vi "Configure_Transfer_SMUs.vi"(6 "Var2 step settings":T3, 8 "error in (no error)":errorcluster, 9 "Var1 sweep settings":T2, 10 "SMU Config":T1, 11 "VISA In":refnum<visa-resource-name>) -> (0 "error out":errorcluster, 3 "VISA Out":refnum<visa-resource-name>)   [LabVIEW 2012]
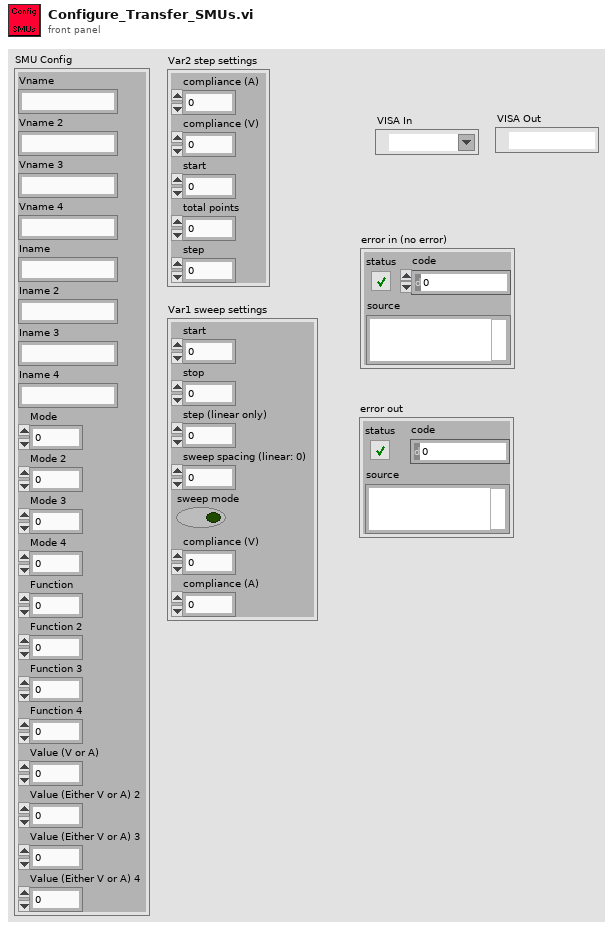
[diagram p1: front panel]
types:
  T1 = cluster{"Vname":string, "Vname 2":string, "Vname 3":string, "Vname 4":string, "Iname":string, "Iname 2":string, "Iname 3":string, "Iname 4":string, "Mode":u16, "Mode 2":u16, "Mode 3":u16, "Mode 4":u16, "Function":u16, "Function 2":u16, "Function 3":u16, "Function 4":u16, "Value (V or A)":dbl, "Value (Either V or A) 2":dbl, "Value (Either V or A) 3":dbl, "Value (Either V or A) 4":dbl}
  T2 = cluster{"start":dbl, "stop":dbl, "step (linear only)":dbl, "sweep spacing (linear: 0)":u16, "sweep mode":bool, "compliance (V)":dbl, "compliance (A)":dbl}
  T3 = cluster{"compliance (A)":dbl, "compliance (V)":dbl, "start":dbl, "total points":u16, "step":dbl}
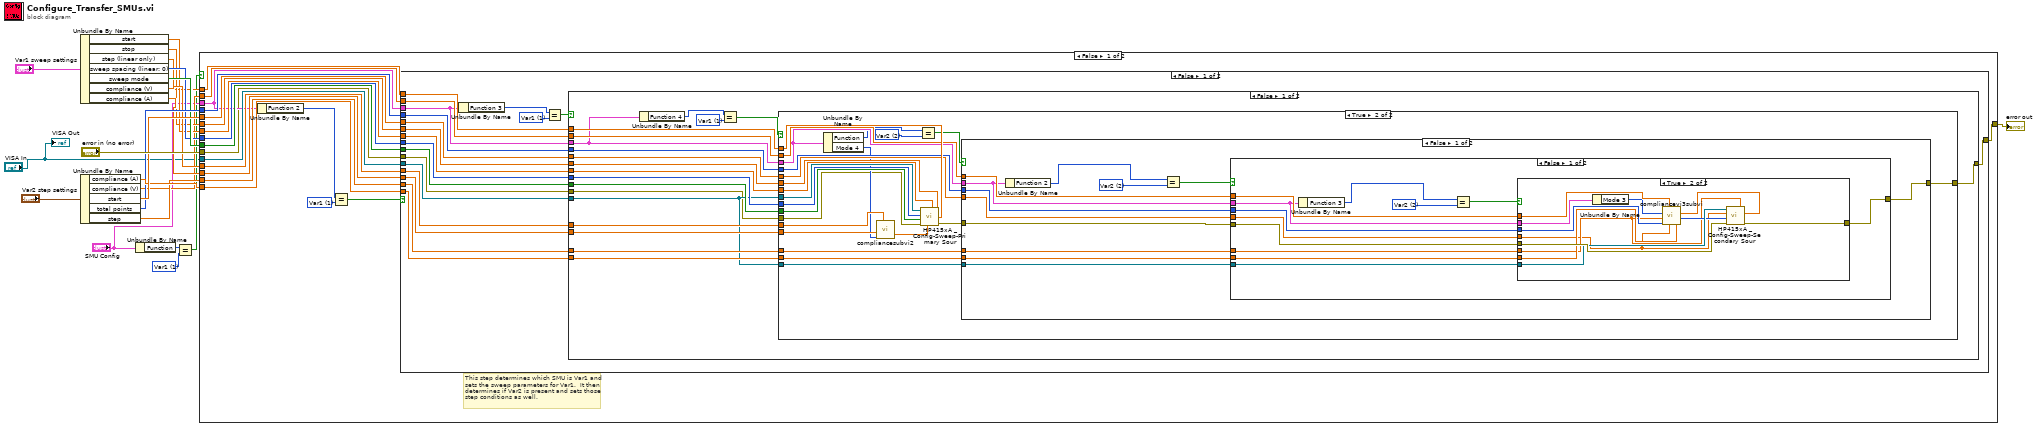
[diagram p0: block diagram]
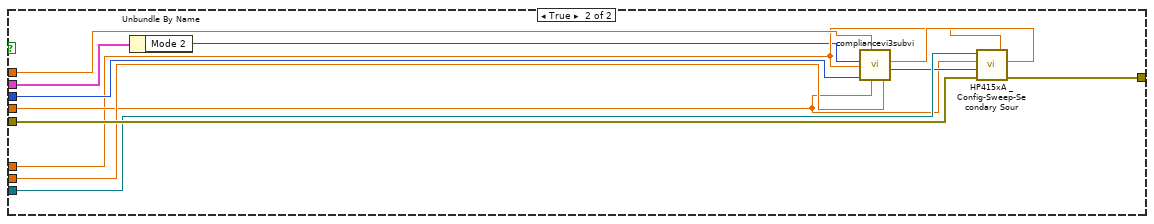
[diagram p4: hidden frame]
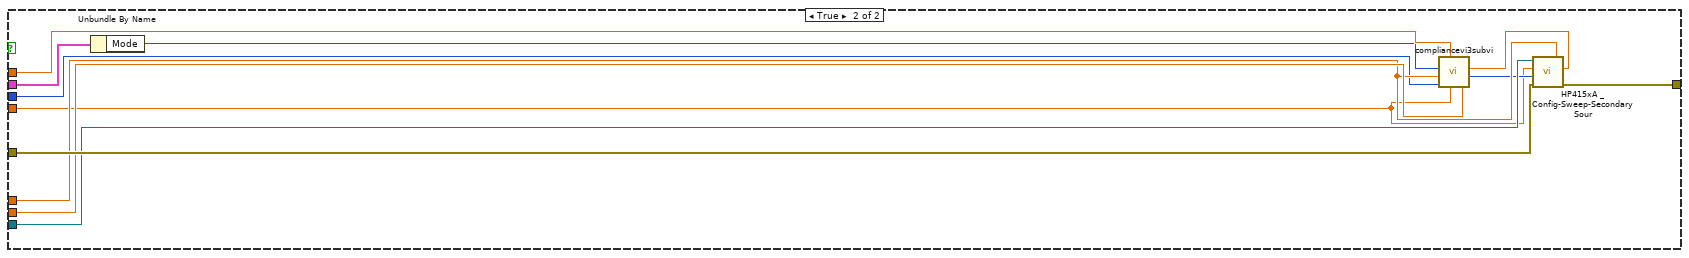
[diagram p5: hidden frame]
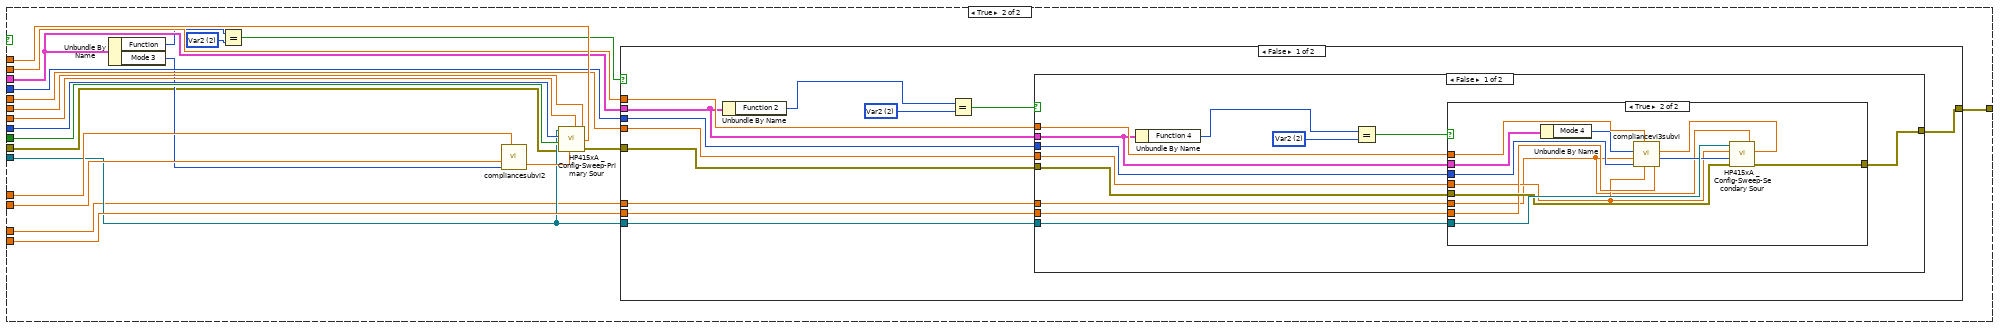
[diagram p6: hidden frame]
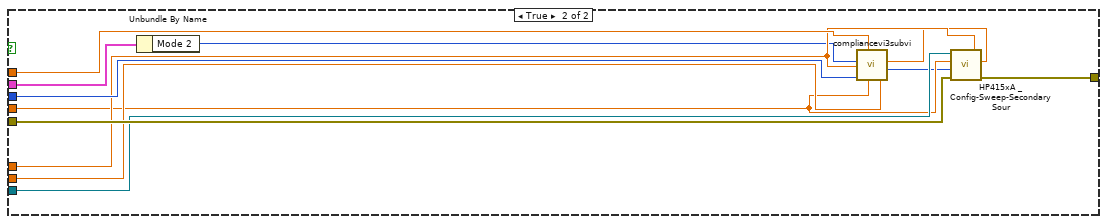
[diagram p8: hidden frame]
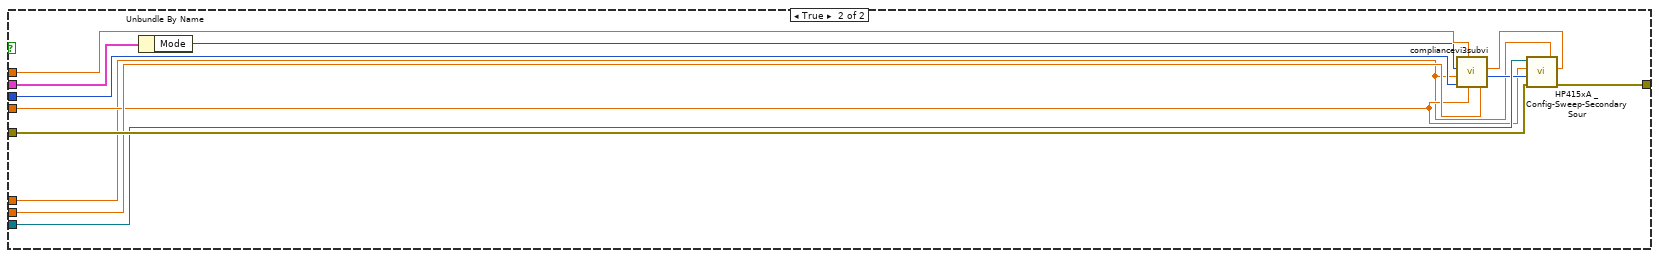
[diagram p9: hidden frame]
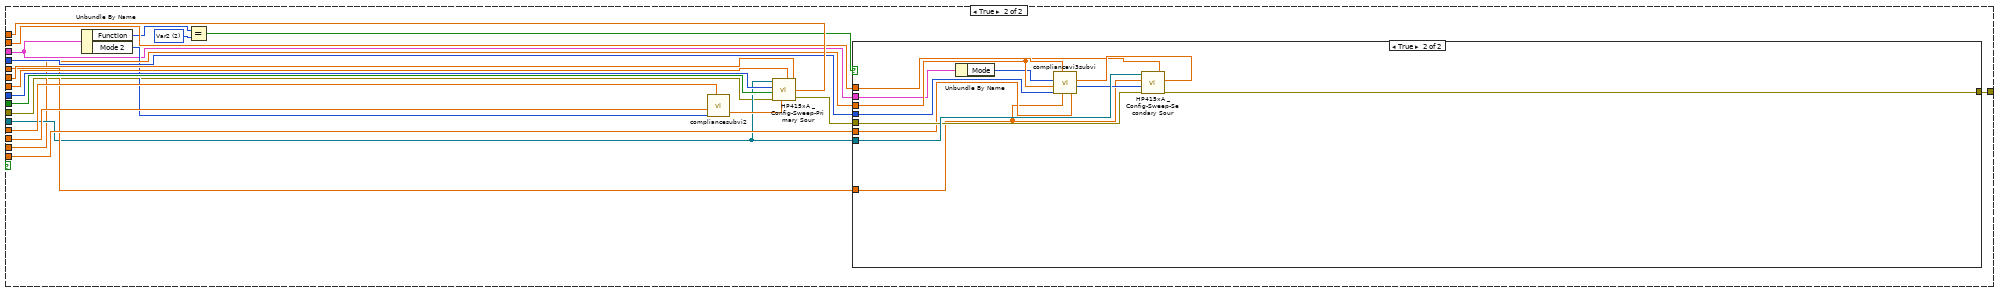
[diagram p10: hidden frame]
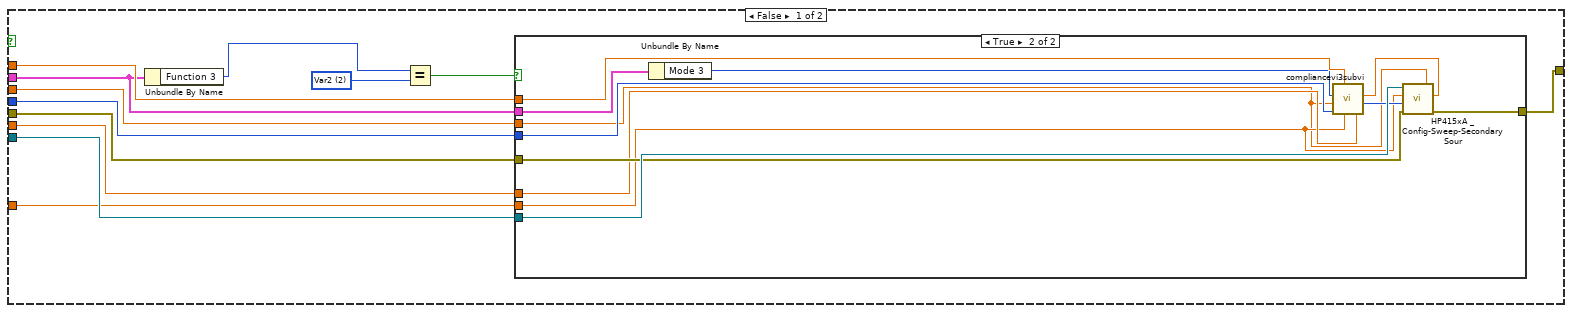
[diagram p11: hidden frame]
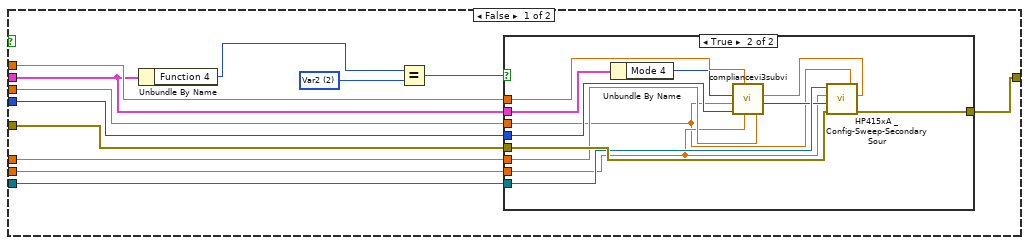
[diagram p12: hidden frame]
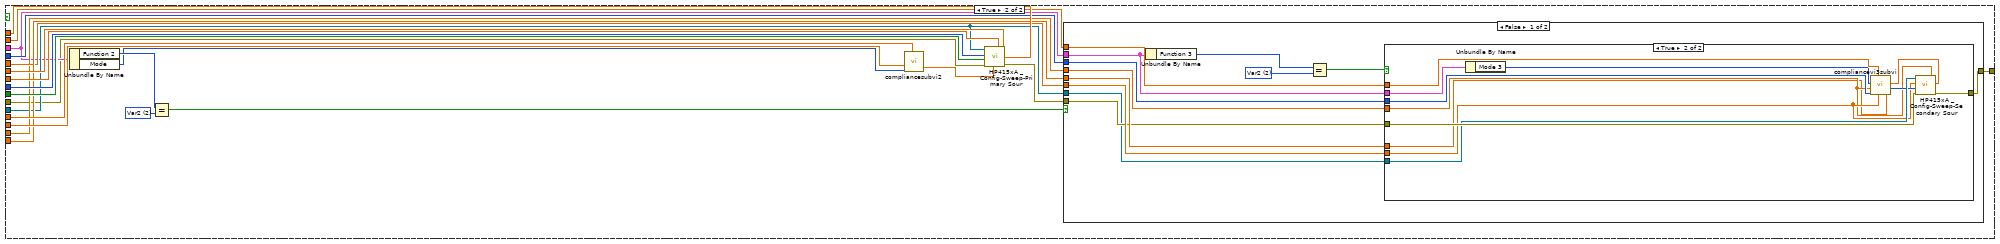
[diagram p14: hidden frame]
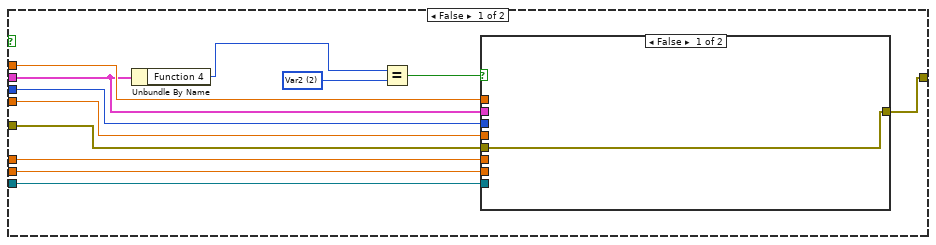
[diagram p15: hidden frame]
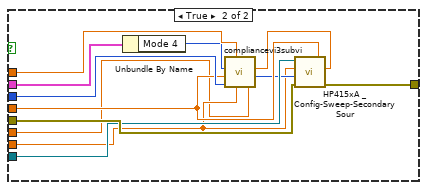
[diagram p16: hidden frame]
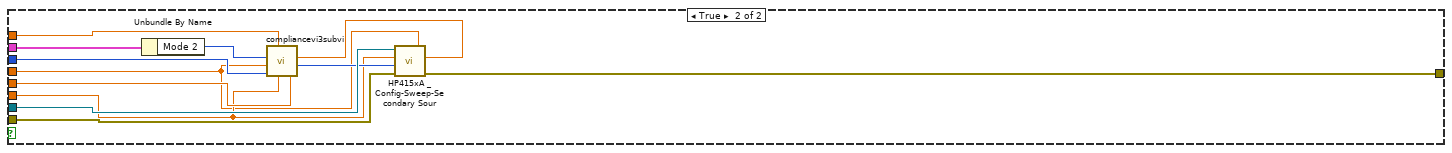
[diagram p17: hidden frame]
diagram:
  w2 = u16 1 items=["disabled", "Var1", "Var2", "Var1'", "Constant"] ("Function")
  n1 = Unbundle By Name("Var1 sweep settings") -> ("start"=w11:dbl, "stop"=w10:dbl, "step (linear only)"=w7:dbl, "sweep spacing (linear: 0)"=w12:u16, "sweep mode"=w13:bool, "compliance (V)"=w14:dbl, "compliance (A)"=w15:dbl)
  n2 = Unbundle By Name("Var2 step settings") -> ("compliance (A)"=w18:dbl, "compliance (V)"=w9:dbl, "start"=w19:dbl, "total points"=w16:u16, "step"=w17:dbl)
  n3 = Unbundle By Name("SMU Config") -> ("Function"=w4:u16)
  n4 = Equal?(x=w4, y=w2) -> (x = y?=w3:bool)
  n5 = case shown="False" w3 {
    tunnel: w14 -> [w38 w350]
    tunnel: w15 -> [w39 w349]
    tunnel: w12 -> [w36 w348]
    tunnel: w13 -> [w37 w347]
    tunnel: w7 -> [w33 w346]
    tunnel: w10 -> [w32 w345]
    tunnel: w11 -> [w34 w344]
    tunnel: "VISA In" -> [w35 w335]
    tunnel: w18 -> [w30 w341]
    tunnel: w9 -> [w29 w340]
    tunnel: w19 -> [w28 w339]
    tunnel: w16 -> [w27 w338]
    tunnel: w17 -> [w26 w337]
    tunnel: "SMU Config" -> [w25 w332]
    tunnel: [w23 w331] -> w20
    tunnel: "error in (no error)" -> [w22 w330]
    frame False {
      w40 = u16 1 items=["disabled", "Var1", "Var2", "Var1'", "Constant"] ("Function")
      # "This step determines which SMU is Var1 and\nsets the sweep parameters for Var1.  It then\ndetermines if Var2 is present and sets those\nstep conditions as well."
      n6 = Unbundle By Name(w25) -> ("Function 2"=w24:u16)
      n7 = Equal?(x=w24, y=w40) -> (x = y?=w31:bool)
      n8 = case shown="False" w31 {
        tunnel: w39 -> [w50 w267]
        tunnel: w38 -> [w51 w266]
        tunnel: w37 -> [w52 w265]
        tunnel: w36 -> [w53 w264]
        tunnel: w35 -> [w57 w255]
        tunnel: w34 -> [w56 w263]
        tunnel: w33 -> [w54 w262]
        tunnel: w32 -> [w55 w261]
        tunnel: w30 -> [w49 w258]
        tunnel: w29 -> [w48 w257]
        tunnel: w28 -> [w46 w256]
        tunnel: w27 -> [w47 w253]
        tunnel: w26 -> [w45 w252]
        tunnel: w25 -> [w44 w249]
        tunnel: [w42 w248] -> w23
        tunnel: w22 -> [w41 w247]
        frame False {
          w59 = u16 1 items=["disabled", "Var1", "Var2", "Var1'", "Constant"] ("Function")
          n9 = Unbundle By Name(w44) -> ("Function 3"=w43:u16)
          n10 = Equal?(x=w43, y=w59) -> (x = y?=w58:bool)
          n11 = case shown="False" w58 {
            tunnel: w57 -> [w64 w171]
            tunnel: w56 -> [w76 w185]
            tunnel: w55 -> [w73 w184]
            tunnel: w54 -> [w72 w183]
            tunnel: w53 -> [w75 w182]
            tunnel: w52 -> [w74 w181]
            tunnel: w51 -> [w71 w180]
            tunnel: w50 -> [w70 w179]
            tunnel: w49 -> [w69 w175]
            tunnel: w48 -> [w68 w174]
            tunnel: w47 -> [w67 w173]
            tunnel: w46 -> [w66 w170]
            tunnel: w45 -> [w65 w169]
            tunnel: w44 -> [w62 w168]
            tunnel: [w61 w165] -> w42
            tunnel: w41 -> [w60 w164]
            frame False {
              w78 = u16 1 items=["disabled", "Var1", "Var2", "Var1'", "Constant"] ("Function")
              n12 = Unbundle By Name(w62) -> ("Function 4"=w63:u16)
              n13 = Equal?(x=w63, y=w78) -> (x = y?=w77:bool)
              n14 = case shown="True" w77 {
                tunnel: w76 -> [_ w101]
                tunnel: w64 -> [_ w100]
                tunnel: w75 -> [_ w99]
                tunnel: w74 -> [_ w98]
                tunnel: w73 -> [_ w97]
                tunnel: w72 -> [_ w96]
                tunnel: w71 -> [_ w95]
                tunnel: w70 -> [_ w94]
                tunnel: w69 -> [_ w91]
                tunnel: w68 -> [_ w90]
                tunnel: w67 -> [_ w89]
                tunnel: w66 -> [_ w88]
                tunnel: w65 -> [_ w87]
                tunnel: w64 -> [_ w85]
                tunnel: w62 -> [_ w84]
                tunnel: [w79 w81] -> w61
                tunnel: w60 -> [w79 w80]
                frame False {
                }
                frame True {
                  w93 = u16 2 items=["disabled", "Var1", "Var2", "Var1'", "Constant"] ("Function")
                  n15 = Unbundle By Name(w84) -> ("Function"=w83:u16, "Mode 4"=w82:u16)
                  n16 = call "compliancesubvi2.vi"("compliance (V)"=w95, "Mode"=w82, "compliance (A)"=w94) -> ("compliance"=w102:dbl)  [unwired: 3 in, 1 out]
                  n17 = Equal?(x=w83, y=w93) -> (x = y?=w92:bool)
                  n18 = call "HP415xA _Config-Sweep-Primary Sour.vi"("step (linear only)"=w96, "stop"=w97, "start"=w101, "compliance"=w102, "error in (no error)"=w80, "sweep mode"=w98, "sweep spacing (linear: 0)"=w99, "VISA session"=w100) -> ("error out"=w86:errorcluster)  [unwired: 2 in]
                  n19 = case shown="False" w92 {
                    tunnel: w91 -> [w112 w161]
                    tunnel: w90 -> [w111 w156]
                    tunnel: w89 -> [w110 w155]
                    tunnel: w88 -> [w109 w157]
                    tunnel: w87 -> [w108 w160]
                    tunnel: w86 -> [w107 w163]
                    tunnel: w85 -> [w106 w162]
                    tunnel: w84 -> [w104 w154]
                    tunnel: [w103 w152] -> w81
                    frame False {
                      w114 = u16 2 items=["disabled", "Var1", "Var2", "Var1'", "Constant"] ("Function")
                      n20 = Unbundle By Name(w104) -> ("Function 2"=w105:u16)
                      n21 = Equal?(x=w105, y=w114) -> (x = y?=w113:bool)
                      n22 = case shown="False" w113 {
                        tunnel: w112 -> [w124 w148]
                        tunnel: w111 -> [w123 w149]
                        tunnel: w110 -> [w122 w147]
                        tunnel: w109 -> [w121 w145]
                        tunnel: w108 -> [w120 w143]
                        tunnel: w107 -> [w119 w151]
                        tunnel: w106 -> [w118 w150]
                        tunnel: w104 -> [w116 w142]
                        tunnel: [w115 w140] -> w103
                        frame False {
                          w126 = u16 2 items=["disabled", "Var1", "Var2", "Var1'", "Constant"] ("Function")
                          n23 = Unbundle By Name(w116) -> ("Function 3"=w117:u16)
                          n24 = Equal?(x=w117, y=w126) -> (x = y?=w125:bool)
                          n25 = case shown="True" w125 {
                            tunnel: w124 -> [_ w135]
                            tunnel: w123 -> [_ w136]
                            tunnel: w122 -> [_ w137]
                            tunnel: w121 -> [_ w131]
                            tunnel: w120 -> [_ w132]
                            tunnel: w119 -> [w127 w139]
                            tunnel: w118 -> [_ w138]
                            tunnel: w116 -> [_ w130]
                            tunnel: [w127 w128] -> w115
                            frame False {
                            }
                            frame True {
                              n26 = Unbundle By Name(w130) -> ("Mode 3"=w129:u16)
                              n27 = call "compliancevi3subvi.vi"("compliance (A)"=w135, "start"=w131, "compliance (V)"=w136, "total points"=w137, "step"=w132, "Mode"=w129) -> ("total points 2"=w134:u16, "compliance"=w133:dbl)  [unwired: 1 in, 1 out]
                              n28 = call "HP415xA _Config-Sweep-Secondary Sour.vi"("compliance"=w133, "step"=w132, "error in (no error)"=w139, "total points"=w134, "start"=w131, "VISA session"=w138) -> ("error out"=w128:errorcluster)  [unwired: 1 in]
                            }
                          }
                        }
                        frame True {
                          n29 = Unbundle By Name(w142) -> ("Mode 2"=w141:u16)
                          n30 = call "compliancevi3subvi.vi"("compliance (A)"=w148, "start"=w145, "compliance (V)"=w149, "total points"=w147, "step"=w143, "Mode"=w141) -> ("total points 2"=w146:u16, "compliance"=w144:dbl)  [unwired: 1 in, 1 out]
                          n31 = call "HP415xA _Config-Sweep-Secondary Sour.vi"("compliance"=w144, "step"=w143, "error in (no error)"=w151, "total points"=w146, "start"=w145, "VISA session"=w150) -> ("error out"=w140:errorcluster)  [unwired: 1 in]
                        }
                      }
                    }
                    frame True {
                      n32 = Unbundle By Name(w154) -> ("Mode"=w153:u16)
                      n33 = call "compliancevi3subvi.vi"("compliance (A)"=w161, "start"=w157, "compliance (V)"=w156, "total points"=w155, "step"=w160, "Mode"=w153) -> ("total points 2"=w158:u16, "compliance"=w159:dbl)  [unwired: 1 in, 1 out]
                      n34 = call "HP415xA _Config-Sweep-Secondary Sour.vi"("compliance"=w159, "step"=w160, "error in (no error)"=w163, "total points"=w158, "start"=w157, "VISA session"=w162) -> ("error out"=w152:errorcluster)  [unwired: 1 in]
                    }
                  }
                }
              }
            }
            frame True {
              w177 = u16 2 items=["disabled", "Var1", "Var2", "Var1'", "Constant"] ("Function")
              n35 = Unbundle By Name(w168) -> ("Function"=w167:u16, "Mode 3"=w166:u16)
              n36 = Equal?(x=w167, y=w177) -> (x = y?=w176:bool)
              n37 = call "compliancesubvi2.vi"("compliance (V)"=w180, "Mode"=w166, "compliance (A)"=w179) -> ("compliance"=w178:dbl)  [unwired: 3 in, 1 out]
              n38 = call "HP415xA _Config-Sweep-Primary Sour.vi"("step (linear only)"=w183, "stop"=w184, "start"=w185, "compliance"=w178, "error in (no error)"=w164, "sweep mode"=w181, "sweep spacing (linear: 0)"=w182, "VISA session"=w171) -> ("error out"=w172:errorcluster)  [unwired: 2 in]
              n39 = case shown="False" w176 {
                tunnel: w175 -> [w193 w244]
                tunnel: w174 -> [w192 w243]
                tunnel: w173 -> [w190 w242]
                tunnel: w172 -> [w195 w246]
                tunnel: w171 -> [w194 w245]
                tunnel: w170 -> [w189 w239]
                tunnel: w169 -> [w191 w238]
                tunnel: w168 -> [w188 w237]
                tunnel: [w186 w235] -> w165
                frame False {
                  w197 = u16 2 items=["disabled", "Var1", "Var2", "Var1'", "Constant"] ("Function")
                  n40 = Unbundle By Name(w188) -> ("Function 2"=w187:u16)
                  n41 = Equal?(x=w187, y=w197) -> (x = y?=w196:bool)
                  n42 = case shown="False" w196 {
                    tunnel: w195 -> [w207 w234]
                    tunnel: w194 -> [w206 w233]
                    tunnel: w193 -> [w205 w230]
                    tunnel: w192 -> [w204 w231]
                    tunnel: w191 -> [w201 w229]
                    tunnel: w190 -> [w203 w232]
                    tunnel: w189 -> [w202 w228]
                    tunnel: w188 -> [w199 w225]
                    tunnel: [w198 w223] -> w186
                    frame False {
                      w209 = u16 2 items=["disabled", "Var1", "Var2", "Var1'", "Constant"] ("Function")
                      n43 = Unbundle By Name(w199) -> ("Function 4"=w200:u16)
                      n44 = Equal?(x=w200, y=w209) -> (x = y?=w208:bool)
                      n45 = case shown="True" w208 {
                        tunnel: w207 -> [w210 w221]
                        tunnel: w206 -> [_ w222]
                        tunnel: w205 -> [_ w219]
                        tunnel: w204 -> [_ w220]
                        tunnel: w203 -> [_ w218]
                        tunnel: w202 -> [_ w215]
                        tunnel: w201 -> [_ w214]
                        tunnel: w199 -> [_ w213]
                        tunnel: [w210 w211] -> w198
                        frame False {
                        }
                        frame True {
                          n46 = Unbundle By Name(w213) -> ("Mode 4"=w212:u16)
                          n47 = call "compliancevi3subvi.vi"("compliance (A)"=w219, "start"=w215, "compliance (V)"=w220, "total points"=w218, "step"=w214, "Mode"=w212) -> ("total points 2"=w217:u16, "compliance"=w216:dbl)  [unwired: 1 in, 1 out]
                          n48 = call "HP415xA _Config-Sweep-Secondary Sour.vi"("compliance"=w216, "step"=w214, "error in (no error)"=w221, "total points"=w217, "start"=w215, "VISA session"=w222) -> ("error out"=w211:errorcluster)  [unwired: 1 in]
                        }
                      }
                    }
                    frame True {
                      n49 = Unbundle By Name(w225) -> ("Mode 2"=w224:u16)
                      n50 = call "compliancevi3subvi.vi"("compliance (A)"=w230, "start"=w228, "compliance (V)"=w231, "total points"=w232, "step"=w229, "Mode"=w224) -> ("total points 2"=w227:u16, "compliance"=w226:dbl)  [unwired: 1 in, 1 out]
                      n51 = call "HP415xA _Config-Sweep-Secondary Sour.vi"("compliance"=w226, "step"=w229, "error in (no error)"=w234, "total points"=w227, "start"=w228, "VISA session"=w233) -> ("error out"=w223:errorcluster)  [unwired: 1 in]
                    }
                  }
                }
                frame True {
                  n52 = Unbundle By Name(w237) -> ("Mode"=w236:u16)
                  n53 = call "compliancevi3subvi.vi"("compliance (A)"=w244, "start"=w239, "compliance (V)"=w243, "total points"=w242, "step"=w238, "Mode"=w236) -> ("total points 2"=w241:u16, "compliance"=w240:dbl)  [unwired: 1 in, 1 out]
                  n54 = call "HP415xA _Config-Sweep-Secondary Sour.vi"("compliance"=w240, "step"=w238, "error in (no error)"=w246, "total points"=w241, "start"=w239, "VISA session"=w245) -> ("error out"=w235:errorcluster)  [unwired: 1 in]
                }
              }
            }
          }
        }
        frame True {
          w260 = u16 2 items=["disabled", "Var1", "Var2", "Var1'", "Constant"] ("Function")
          n55 = Unbundle By Name(w249) -> ("Function"=w251:u16, "Mode 2"=w250:u16)
          n56 = Equal?(x=w251, y=w260) -> (x = y?=w259:bool)
          n57 = call "compliancesubvi2.vi"("compliance (V)"=w266, "Mode"=w250, "compliance (A)"=w267) -> ("compliance"=w268:dbl)  [unwired: 3 in, 1 out]
          n58 = call "HP415xA _Config-Sweep-Primary Sour.vi"("step (linear only)"=w262, "stop"=w261, "start"=w263, "compliance"=w268, "error in (no error)"=w247, "sweep mode"=w265, "sweep spacing (linear: 0)"=w264, "VISA session"=w255) -> ("error out"=w254:errorcluster)  [unwired: 2 in]
          n59 = case shown="True" w259 {
            tunnel: w258 -> [w277 w326]
            tunnel: w257 -> [w276 w325]
            tunnel: w256 -> [w274 w321]
            tunnel: w255 -> [w279 w329]
            tunnel: w254 -> [w273 w328]
            tunnel: w253 -> [w275 w327]
            tunnel: w252 -> [w272 w323]
            tunnel: w249 -> [w271 w320]
            tunnel: [w269 w318] -> w248
            frame False {
              w280 = u16 2 items=["disabled", "Var1", "Var2", "Var1'", "Constant"] ("Function")
              n60 = Unbundle By Name(w271) -> ("Function 3"=w270:u16)
              n61 = Equal?(x=w270, y=w280) -> (x = y?=w278:bool)
              n62 = case shown="True" w278 {
                tunnel: w279 -> [w289 w317]
                tunnel: w277 -> [w288 w315]
                tunnel: w276 -> [w286 w313]
                tunnel: w275 -> [w287 w314]
                tunnel: w274 -> [w284 w311]
                tunnel: w273 -> [w290 w316]
                tunnel: w272 -> [w285 w309]
                tunnel: w271 -> [w283 w308]
                tunnel: [w281 w306] -> w269
                frame False {
                  w292 = u16 2 items=["disabled", "Var1", "Var2", "Var1'", "Constant"] ("Function")
                  n63 = Unbundle By Name(w283) -> ("Function 4"=w282:u16)
                  n64 = Equal?(x=w282, y=w292) -> (x = y?=w291:bool)
                  n65 = case shown="True" w291 {
                    tunnel: w290 -> [w293 w305]
                    tunnel: w289 -> [_ w304]
                    tunnel: w288 -> [_ w302]
                    tunnel: w287 -> [_ w303]
                    tunnel: w286 -> [_ w301]
                    tunnel: w285 -> [_ w298]
                    tunnel: w284 -> [_ w299]
                    tunnel: w283 -> [_ w296]
                    tunnel: [w293 w294] -> w281
                    frame False {
                    }
                    frame True {
                      n66 = Unbundle By Name(w296) -> ("Mode 4"=w295:u16)
                      n67 = call "compliancevi3subvi.vi"("compliance (A)"=w302, "start"=w299, "compliance (V)"=w301, "total points"=w303, "step"=w298, "Mode"=w295) -> ("total points 2"=w300:u16, "compliance"=w297:dbl)  [unwired: 1 in, 1 out]
                      n68 = call "HP415xA _Config-Sweep-Secondary Sour.vi"("compliance"=w297, "step"=w298, "error in (no error)"=w305, "total points"=w300, "start"=w299, "VISA session"=w304) -> ("error out"=w294:errorcluster)  [unwired: 1 in]
                    }
                  }
                }
                frame True {
                  n69 = Unbundle By Name(w308) -> ("Mode 3"=w307:u16)
                  n70 = call "compliancevi3subvi.vi"("compliance (A)"=w315, "start"=w311, "compliance (V)"=w313, "total points"=w314, "step"=w309, "Mode"=w307) -> ("total points 2"=w312:u16, "compliance"=w310:dbl)  [unwired: 1 in, 1 out]
                  n71 = call "HP415xA _Config-Sweep-Secondary Sour.vi"("compliance"=w310, "step"=w309, "error in (no error)"=w316, "total points"=w312, "start"=w311, "VISA session"=w317) -> ("error out"=w306:errorcluster)  [unwired: 1 in]
                }
              }
            }
            frame True {
              n72 = Unbundle By Name(w320) -> ("Mode"=w319:u16)
              n73 = call "compliancevi3subvi.vi"("compliance (A)"=w326, "start"=w321, "compliance (V)"=w325, "total points"=w327, "step"=w323, "Mode"=w319) -> ("total points 2"=w322:u16, "compliance"=w324:dbl)  [unwired: 1 in, 1 out]
              n74 = call "HP415xA _Config-Sweep-Secondary Sour.vi"("compliance"=w324, "step"=w323, "error in (no error)"=w328, "total points"=w322, "start"=w321, "VISA session"=w329) -> ("error out"=w318:errorcluster)  [unwired: 1 in]
            }
          }
        }
      }
    }
    frame True {
      w343 = u16 2 items=["disabled", "Var1", "Var2", "Var1'", "Constant"] ("Function 2")
      n75 = Unbundle By Name(w332) -> ("Function 2"=w334:u16, "Mode"=w333:u16)
      n76 = Equal?(x=w334, y=w343) -> (x = y?=w342:bool)
      n77 = call "compliancesubvi2.vi"("compliance (V)"=w350, "Mode"=w333, "compliance (A)"=w349) -> ("compliance"=w351:dbl)  [unwired: 3 in, 1 out]
      n78 = call "HP415xA _Config-Sweep-Primary Sour.vi"("step (linear only)"=w346, "stop"=w345, "start"=w344, "compliance"=w351, "error in (no error)"=w330, "sweep mode"=w347, "sweep spacing (linear: 0)"=w348, "VISA session"=w335) -> ("error out"=w336:errorcluster)  [unwired: 2 in]
      n79 = case shown="False" w342 {
        tunnel: w341 -> [w360 w410]
        tunnel: w340 -> [w361 w409]
        tunnel: w339 -> [w358 w406]
        tunnel: w338 -> [w359 w408]
        tunnel: w337 -> [w357 w404]
        tunnel: w336 -> [w356 w412]
        tunnel: w335 -> [w355 w411]
        tunnel: w332 -> [w353 w403]
        tunnel: [w352 w401] -> w331
        frame False {
          w363 = u16 2 items=["disabled", "Var1", "Var2", "Var1'", "Constant"] ("Function 2")
          n80 = Unbundle By Name(w353) -> ("Function 3"=w354:u16)
          n81 = Equal?(x=w354, y=w363) -> (x = y?=w362:bool)
          n82 = case shown="True" w362 {
            tunnel: w361 -> [w371 w392]
            tunnel: w360 -> [w372 w393]
            tunnel: w359 -> [w369 w398]
            tunnel: w358 -> [w370 w395]
            tunnel: w357 -> [w368 w394]
            tunnel: w356 -> [w373 w400]
            tunnel: w355 -> [w367 w399]
            tunnel: w353 -> [w365 w391]
            tunnel: [w364 w389] -> w352
            frame False {
              w375 = u16 2 items=["disabled", "Var1", "Var2", "Var1'", "Constant"] ("Function 2")
              n83 = Unbundle By Name(w365) -> ("Function 4"=w366:u16)
              n84 = Equal?(x=w366, y=w375) -> (x = y?=w374:bool)
              n85 = case shown="False" w374 {
                tunnel: w373 -> [w376 w388]
                tunnel: w372 -> [_ w380]
                tunnel: w371 -> [_ w381]
                tunnel: w370 -> [_ w382]
                tunnel: w369 -> [_ w386]
                tunnel: w368 -> [_ w384]
                tunnel: w367 -> [_ w387]
                tunnel: w365 -> [_ w379]
                tunnel: [w376 w377] -> w364
                frame False {
                }
                frame True {
                  n86 = Unbundle By Name(w379) -> ("Mode 4"=w378:u16)
                  n87 = call "compliancevi3subvi.vi"("compliance (A)"=w380, "start"=w382, "compliance (V)"=w381, "total points"=w386, "step"=w384, "Mode"=w378) -> ("total points 2"=w383:u16, "compliance"=w385:dbl)  [unwired: 1 in, 1 out]
                  n88 = call "HP415xA _Config-Sweep-Secondary Sour.vi"("compliance"=w385, "step"=w384, "error in (no error)"=w388, "total points"=w383, "start"=w382, "VISA session"=w387) -> ("error out"=w377:errorcluster)  [unwired: 1 in]
                }
              }
            }
            frame True {
              n89 = Unbundle By Name(w391) -> ("Mode 3"=w390:u16)
              n90 = call "compliancevi3subvi.vi"("compliance (A)"=w393, "start"=w395, "compliance (V)"=w392, "total points"=w398, "step"=w394, "Mode"=w390) -> ("total points 2"=w397:u16, "compliance"=w396:dbl)  [unwired: 1 in, 1 out]
              n91 = call "HP415xA _Config-Sweep-Secondary Sour.vi"("compliance"=w396, "step"=w394, "error in (no error)"=w400, "total points"=w397, "start"=w395, "VISA session"=w399) -> ("error out"=w389:errorcluster)  [unwired: 1 in]
            }
          }
        }
        frame True {
          n92 = Unbundle By Name(w403) -> ("Mode 2"=w402:u16)
          n93 = call "compliancevi3subvi.vi"("compliance (A)"=w410, "start"=w406, "compliance (V)"=w409, "total points"=w408, "step"=w404, "Mode"=w402) -> ("total points 2"=w407:u16, "compliance"=w405:dbl)  [unwired: 1 in, 1 out]
          n94 = call "HP415xA _Config-Sweep-Secondary Sour.vi"("compliance"=w405, "step"=w404, "error in (no error)"=w412, "total points"=w407, "start"=w406, "VISA session"=w411) -> ("error out"=w401:errorcluster)  [unwired: 1 in]
        }
      }
    }
  }
  "error out" <- w20
  "VISA Out" <- "VISA In"
